vi "Creators Created Queues.vi"(8 "Created Queue Alias":string, 9 "Priority?":bool, 10 "Msg Strategy":refnum<class "Msg Strategy.lvclass">, 11 "TEMPLATE Event in":refnum<class "TEMPLATE Event.lvclass">) -> (3 "TEMPLATE Event out":refnum<class "TEMPLATE Event.lvclass">)   [LabVIEW 2021, in "_Template.lvlib" / "Templates.lvlib" / "TEMPLATE Event.lvlib" / "TEMPLATE Event.lvclass"]
uses:
  TEMPLATE Event.lvclass
  <vilib>/Nathan Davis/jettl/jettl/Msg Strategy/Msg Strategy.lvclass
  TEMPLATE Event.lvclass/TEMPLATE Event.ctl
  <vilib>/Nathan Davis/jettl/jettl/Event/Event.lvclass
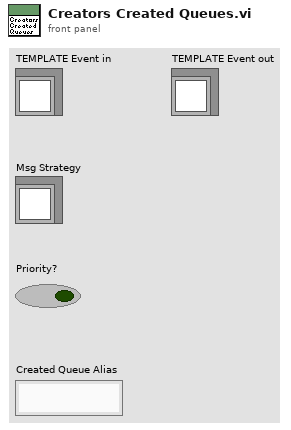
[diagram p1: front panel]
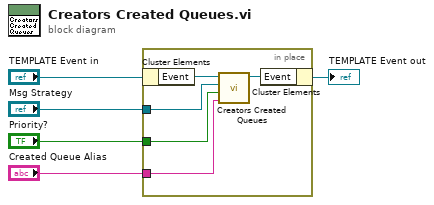
[diagram p0: block diagram]
diagram:
  n1 = in-place {
    in-place-border: "Msg Strategy" -> [w8]
    in-place-border: "Priority?" -> [w7]
    in-place-border: "Created Queue Alias" -> [w6]
    n2 = in-place-cluster #1("TEMPLATE Event in") -> ("Event"=w10:refnum<class "Event.lvclass">)
    n3 = call-dynamic "Creators Created Queues.vi"("Created Queue Alias"=w6, "Priority?"=w7, "Msg Strategy"=w8, "Event in"=w10) -> ("Event out"=w9:refnum<class "Event.lvclass">)  [unwired: 7 in]
    n4 = in-place-cluster #1("Event"=w9) -> (→"TEMPLATE Event out":refnum<class "TEMPLATE Event.lvclass">)
  }
